vi "test--changes.vi"() -> ()   [LabVIEW 2021]
doc: "test VI for looking at changes applied.\n\n<b>Code Developed By:</b>\nTechnology Service Corporation\nwww.tsc.com/atcs\n\nDeveloper:\nDaniel Coons"
uses:
  material--ppl--target.lvlibp/main.vi
  src/Material Theme/Material Theme.lvclass
  material--ppl--target.lvlibp
panel:
  in  "Save?":bool
  in  "Open Front Panel?":bool
  out "error out":errorcluster
  in  "Test UI":u16(ring) items=["UI Test--the--Theme", "Example UI", "Sandbox Test UI", "UI Plot Update", "System Controls", "PPL--Test"]
  in  "Theme":u16(ring) items=["Light", "Light Medium Contrast", "Light High Contrast", "Dark", "Dark Medium Contrast", "Dark High Contrast"]
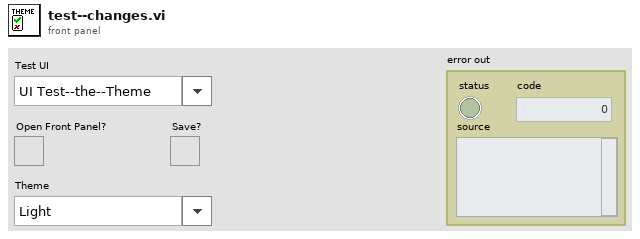
[diagram p1: front panel]
types:
  T1 = enum32{"Invalid", "Standard", "Closed", "Hidden", "Minimized", "Maximized"}
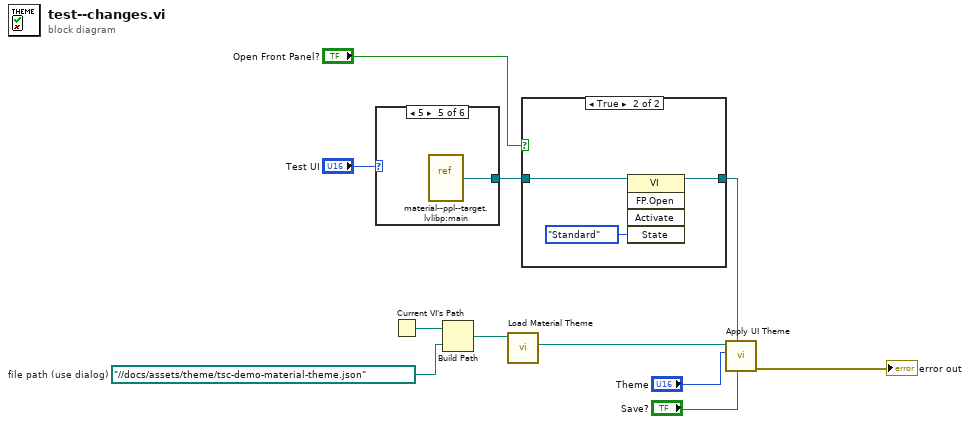
[diagram p0: block diagram]
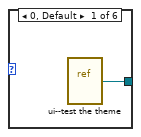
[diagram p3: hidden frame]
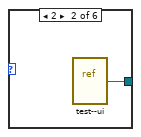
[diagram p4: hidden frame]
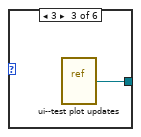
[diagram p5: hidden frame]
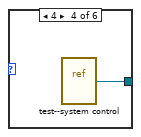
[diagram p6: hidden frame]
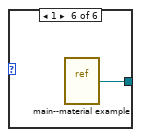
[diagram p7: hidden frame]
diagram:
  w10 = path "../../docs/assets/theme/tsc-demo-material-theme.json"  # file path (use dialog)
  n1 = case shown="5" "Test UI" {
    tunnel: [w12 w13 w14 w15 w16 w17] -> w7
    frame 0, Default {
      n2 = vi-ref "ui--test the theme.vi"() -> (w12:refnum<vi>)
    }
    frame 2 {
      n3 = vi-ref "test--ui.vi"() -> (w13:refnum<vi>)
    }
    frame 3 {
      n4 = vi-ref "ui--test plot updates.vi"() -> (w14:refnum<vi>)
    }
    frame 4 {
      n5 = vi-ref "test--system control.vi"() -> (w15:refnum<vi>)
    }
    frame 5 {
      n6 = vi-ref "material--ppl--target.lvlibp:main.vi"() -> (w16:refnum<vi>)
    }
    frame 1 {
      n7 = vi-ref "main--material example.vi"() -> (w17:refnum<vi>)
    }
  }
  n8 = Current VI's Path() -> (path=w11:path)
  n9 = Build Path(base path=w11, name or relative path=w10) -> (appended path=w9:path)
  n10 = call "Load Material Theme.vi"("file path"=w9) -> ("Theme"=w4:refnum<class "Material Theme.lvclass">)  [unwired: 8 in, 2 out]
  n11 = case shown="True" "Open Front Panel?" {
    tunnel: w7 -> [w18 w21]
    tunnel: [w18 w20] -> w5
    frame False {
    }
    frame True {
      n12 = invoke class="VI" method="FP.Open"(reference=w21, "State"=T1."Standard") -> (reference out=w20:refnum<vi>)  [unwired: 3 in, 4 out]
    }
  }
  n13 = call "Apply UI Theme.vi"("save?"="Save?", "VI Refnum"=w5, "Theme Mode"="Theme", "Material Theme in"=w4) -> ("error out"=→"error out":errorcluster)  [unwired: 6 in, 1 out]
